vi "Simulate.vi"(0 "error in":errorcluster, 5 "Telnet":refnum<k24>, 7 "port":i32(ring) items=["DIN", "DOUT", "RDO", "OPOUT", "TPOUT", "WDI", "WDO", "AIN", "AOUT", "GIN", "GOUT"], 9 "index":i32, 11 "value":i32) -> (4 "error out":errorcluster, 6 "KclCommand":string, 10 "Succeed":bool, 15 "ErrorText":string)   [LabVIEW 2018, in "UnderAutomation.Fanuc.lvlib"]
uses:
  UnderAutomation.Fanuc.lvlib
  C:/Users/fg/Documents/Fanuc.vi/LabVIEW_2024/UnderAutomation.Fanuc/lib/UnderAutomation.Fanuc.dll
  LabVIEW_2024/UnderAutomation.Fanuc/lib/UnderAutomation.Fanuc.dll
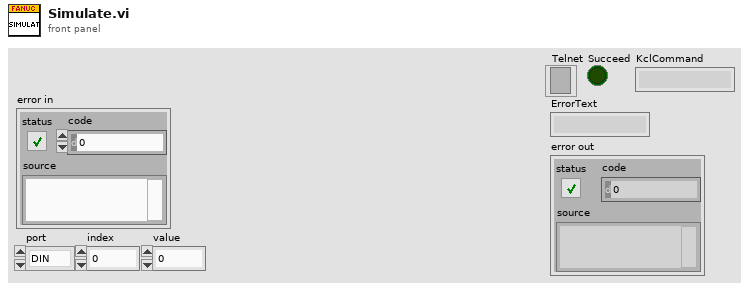
[diagram p1: front panel]
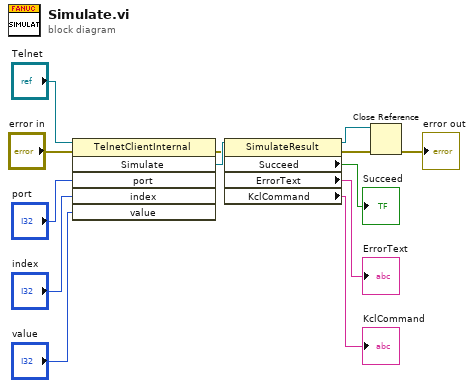
[diagram p0: block diagram]
diagram:
  n1 = invoke class="TelnetClientInternal" method="Simulate"(reference="Telnet", error in="error in", "port"="port", "index"="index", "value"="value") -> (error out=w8:errorcluster, "Simulate"=w11:refnum<k24>)  [unwired: 1 in, 4 out]
  n2 = property class="SimulateResult"(reference=w11, error in=w8) -> (reference out=w4:refnum<k24>, error out=w5:errorcluster, "Succeed"=→"Succeed":bool, "ErrorText"=→"ErrorText":string, "KclCommand"=→"KclCommand":string)
  n3 = Close Reference(reference=w4, error in (no error)=w5) -> (error out=→"error out":errorcluster)
